vi "main.vi"() -> ()   [LabVIEW 2014]
uses:
  <vilib>/Instr/_visa.llb/VISA Configure Serial Port (Instr).vi
  <instrlib>/Keithley 24XX/Public/Data/Read (Single Point).vi
  <instrlib>/Keithley 24XX/Keithley 24XX.lvlib
panel:
  in  "Start Button":bool
  in  "Operation Mode":bool
  out "Humidity":sgl
  out "Humidity Data":string
  in  "Humidity Data":path=path "C:/Users/Administrator/Documents/humidity_sensing_setup/data/dumb/data_dumb_2.txt"
  out "Humidity Data Graph":sgl(graph)=5460.51
  out "Resistance Data":string
  in  "Resistance Data":path=path "C:/Users/Administrator/Documents/humidity_sensing_setup/data/dumb/data_dumb_1.txt"
  out "Current Data":string
  in  "Current Data":path=path "C:/Users/Administrator/Documents/humidity_sensing_setup/data/dumb/data_dumb.txt"
  in  "Sampling rate (ms/pt)":i32=1000
  in  "Stop Voltage/Current":dbl=1.0
  in  "Start Voltage/Current":dbl=1.0
  in  "current multiplier":dbl=1000000.0
  in  "stop button":bool
  out "Current Data Graph":sgl(graph)=0.0001831192
  out "Resistance Data Graph":sgl(graph)=5460.51
  in  "loop num":dbl=10000000000.0
  in  "Step":dbl
  in  "Source Mode  (0: Voltage)":u16(ring) items=["Voltage", "Current"]
  in  "Compliance  Level (0.1)":dbl=1.0
  in  "Enable Resistance Auto Range (T:Enable)":bool
  in  "Enable Current Auto Range (T:Enable)":bool=TRUE
  in  "Enable Voltage Auto Range (T:Enable)":bool
  in  "Resistance Manual Range (1.0)":dbl=1.0
  in  "Current Manual Range (1.0)":dbl=1.0
  in  "Voltage Manual Range (1.0)":dbl=1.0
  out "Resistance":sgl
  out "Current":sgl
  out "Voltage":sgl
  in  "Serial Configuration":T1={"Baud Rate"=9600, "Parity"=0, "Data Bits"=8, "Stop Bits"=10, "Flow Control"=0} {"Flow Control" items=["None", "XON/XOFF", "RTS/CTS", "XON/XOFF & RTS/CTS", "DTR/DSR", "XON/XOFF & DTR/DSR"]; "Stop Bits" items=["1.0"=10, "1.5"=15, "2.0"=20]; "Data Bits" items=["7"=7, "8"=8]; "Parity" items=["None", "Odd", "Even", "Mark", "Space"]; "Baud Rate" items=["300"=300, "600"=600, "1200"=1200, "2400"=2400, "4800"=4800, "9600"=9600, "19200"=19200]}
  in  "Keithley VISA resource name":refnum<visa-resource-name>="GPIB9::24::INSTR"
  out "Arduino Status":bool
  out "error out":errorcluster
  in  "error in":errorcluster
  in  "instr name":string="Arduino"
  in  "write":bool
  in  "buffer size":u32=256
  in  "timeout (ms)":u32=10000
  in  "flow control":u16
  in  "stop bits":u16=10
  in  "parity":u16(ring) items=["None", "Odd", "Even", "Mark", "Space"]
  in  "data bits":u16=8 min=5 max=8 step=1
  in  "baud rate":u32=9600
  in  "write string":string
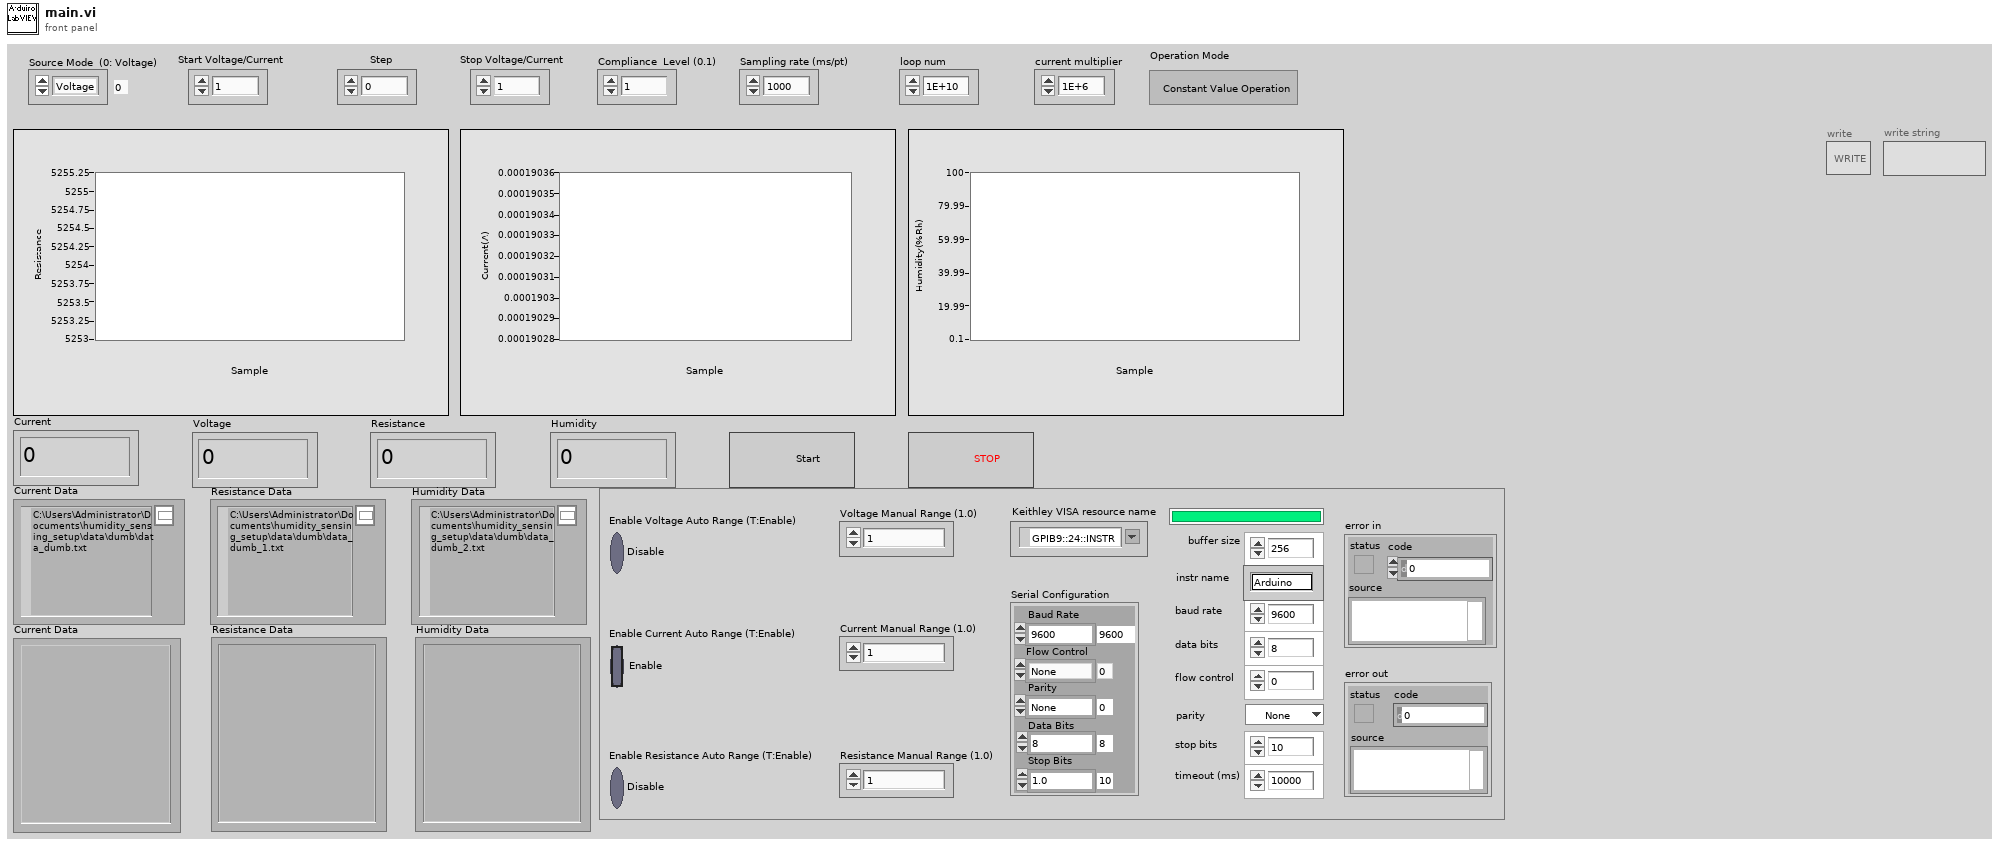
[diagram p1: front panel]
types:
  T1 = cluster{"Baud Rate":u32, "Parity":u16, "Data Bits":u16, "Stop Bits":u16, "Flow Control":u16}
  T2 = enum16{"open", "replace", "create", "open or create", "replace or create", "replace or create with confirmation"}
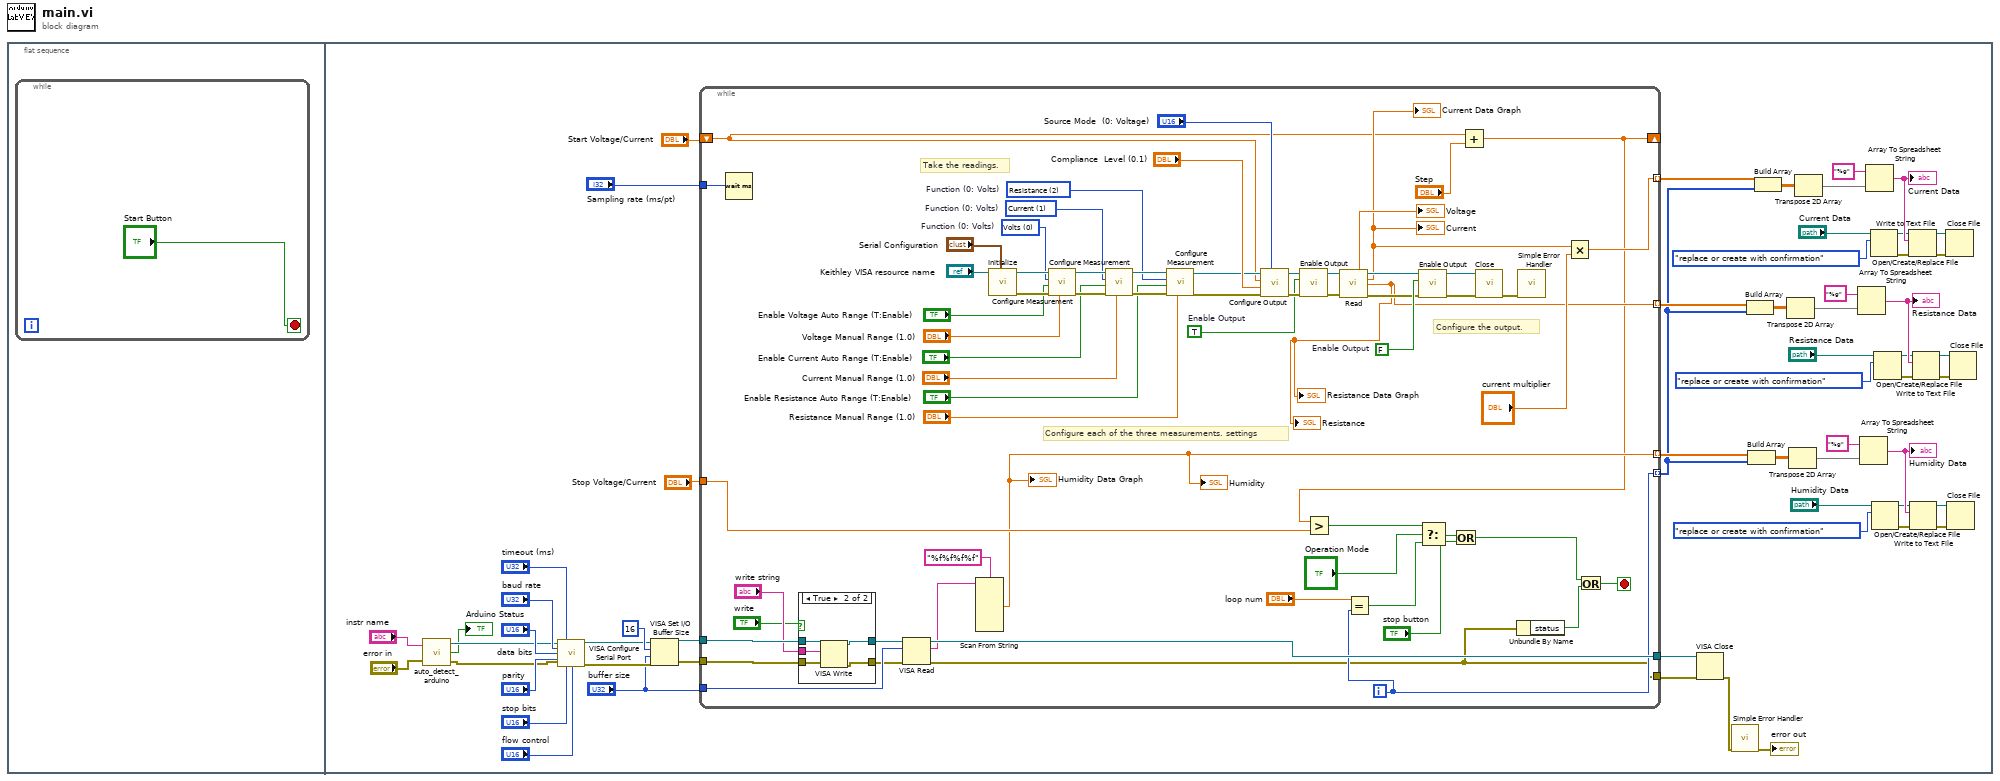
[diagram p0: block diagram]
diagram:
  n1 = flat-sequence {
    frame #0 {
      n2 = while {
        stop <- "Start Button" stop-if-true
      }
    }
    frame #1 {
      n3 = call "auto_detect_arduino.vi"("instr name"="instr name", "error in"="error in") -> ("VISA resource name"=w51:refnum<visa-resource-name>, "status"=→"Arduino Status":bool, "error out"=w50:errorcluster)
      n4 = call-poly "VISA Configure Serial Port"("VISA resource name"=w51, "timeout (10sec)"="timeout (ms)", "baud rate (9600)"="baud rate", "data bits (8)"="data bits", "parity (0:none)"="parity", "error in (no error)"=w50, "stop bits (10: 1 bit)"="stop bits", "flow control (0:none)"="flow control") -> ("VISA resource name out"=w47:refnum<visa-resource-name>, "error out"=w46:errorcluster)  [unwired: 6 in]
      n5 = VISA Set I/O Buffer Size(VISA resource name=w47, mask (16)=u16 16 ("I/O Receive\nBuffer mask"), size (4096)="buffer size", error in (no error)=w46) -> (VISA resource name out=w45:refnum<visa-resource-name>, error out=w44:errorcluster)
      n6 = while {
        tunnel: w45 -> [w120]
        tunnel: w44 -> [w119]
        tunnel: [w121] -> w59
        tunnel: [w63] -> w58
        tunnel: "buffer size" -> [w122]
        tunnel: [w65] -> w3 mode=indexing
        tunnel: "Sampling rate (ms/pt)" -> [w76]
        tunnel: "Stop Voltage/Current" -> [w75]
        tunnel: [w74] -> w16 mode=indexing
        tunnel: [w73] -> w2 mode=indexing
        tunnel: [w72] -> w15 mode=indexing
        shift-right: [w64] -> _
        shift-left: "Start Voltage/Current" -> [w71]
        i -> [w73]
        stop <- w123 stop-if-true
        w85 = TRUE  # Enable Output
        w95 = FALSE  # Enable Output
        w102 = u16 2 items=["Volts", "Current", "Resistance"]  # Function (0: Volts)
        w103 = u16 1 items=["Volts", "Current", "Resistance"]  # Function (0: Volts)
        w104 = u16 0 items=["Volts", "Current", "Resistance"]  # Function (0: Volts)
        # "Take the readings."
        # "Configure the output."
        # "Configure each of the three measurements. settings"
        n7 = Wait (ms)(milliseconds to wait=w76) -> ()  [unwired: 1 out]
        n8 = case shown="True" "write" {
          tunnel: w120 -> [w125 w130]
          tunnel: w119 -> [w124 w129]
          tunnel: [w125 w128] -> w118
          tunnel: [w124 w127] -> w117
          tunnel: "write string" -> [_ w126]
          frame False {
          }
          frame True {
            n9 = VISA Write(VISA resource name=w130, write buffer=w126, error in (no error)=w129) -> (VISA resource name out=w128:refnum<visa-resource-name>, error out=w127:errorcluster)  [unwired: 1 out]
          }
        }
        n10 = VISA Read(VISA resource name=w118, byte count=w122, error in (no error)=w117) -> (VISA resource name out=w121:refnum<visa-resource-name>, read buffer=w60:string, error out=w63:errorcluster)  [unwired: 1 out]
        n11 = Scan From String(format string="%f%f%f%f", input string=w60) -> (output 1=w65:sgl)  [unwired: 9 in, 3 out]
        "Humidity Data Graph" <- w65
        "Humidity" <- w65
        n12 = call <instrlib>:"Initialize.vi"("Serial Configuration"="Serial Configuration", "VISA resource name"="Keithley VISA resource name") -> ("error out"=w109:errorcluster, "VISA resource name out"=w110:refnum<visa-resource-name>)  [unwired: 8 in]
        n13 = call <instrlib>:"Configure Measurement.vi"("Manual Range (1.0)"="Voltage Manual Range (1.0)", "error in (no error)"=w109, "Enable Auto Range (T:Enable)"="Enable Voltage Auto Range (T:Enable)", "Function (0: Volts)"=w104, "VISA resource name"=w110) -> ("error out"=w107:errorcluster, "VISA resource name out"=w108:refnum<visa-resource-name>)  [unwired: 5 in]
        n14 = call <instrlib>:"Configure Measurement.vi"("Manual Range (1.0)"="Current Manual Range (1.0)", "error in (no error)"=w107, "Enable Auto Range (T:Enable)"="Enable Current Auto Range (T:Enable)", "Function (0: Volts)"=w103, "VISA resource name"=w108) -> ("error out"=w106:errorcluster, "VISA resource name out"=w105:refnum<visa-resource-name>)  [unwired: 5 in]
        n15 = call <instrlib>:"Configure Measurement.vi"("Manual Range (1.0)"="Resistance Manual Range (1.0)", "error in (no error)"=w106, "Enable Auto Range (T:Enable)"="Enable Resistance Auto Range (T:Enable)", "Function (0: Volts)"=w102, "VISA resource name"=w105) -> ("error out"=w84:errorcluster, "VISA resource name out"=w83:refnum<visa-resource-name>)  [unwired: 5 in]
        n16 = call <instrlib>:"Configure Output.vi"("Source Mode  (0: Voltage)"="Source Mode  (0: Voltage)", "error in (no error)"=w84, "Compliance  Level (0.1)"="Compliance  Level (0.1)", "Output Level (0)"=w71, "VISA resource name"=w83) -> ("error out"=w86:errorcluster, "VISA resource name out"=w87:refnum<visa-resource-name>)  [unwired: 5 in]
        n17 = call <instrlib>:"Enable Output.vi"("error in (no error)"=w86, "Enable Output (T: Enable)"=w85, "VISA resource name"=w87) -> ("error out"=w89:errorcluster, "VISA resource name out"=w88:refnum<visa-resource-name>)  [unwired: 7 in]
        n18 = call-poly <instrlib>:"Read.vi"("VISA resource name"=w88, "error in (no error)"=w89) -> ("Voltage"=→"Voltage":sgl, "VISA resource name out"=w90:refnum<visa-resource-name>, "Current"=w78:sgl, "Resistance"=w72:sgl, "error out"=w91:errorcluster)  [unwired: 7 in, 2 out]
        "Current" <- w78
        "Resistance" <- w72
        "Resistance Data Graph" <- w72
        "Current Data Graph" <- w78
        n19 = Equal?(x="loop num", y=w73) -> (x = y?=w66:bool)
        n20 = call <instrlib>:"Enable Output.vi"("error in (no error)"=w91, "Enable Output (T: Enable)"=w95, "VISA resource name"=w90) -> ("error out"=w92:errorcluster, "VISA resource name out"=w93:refnum<visa-resource-name>)  [unwired: 7 in]
        n21 = Add(x=w71, y="Step") -> (x+y=w64:dbl)
        n22 = Greater?(x=w64, y=w75) -> (0:w69:bool)
        n23 = Select(t=w69, s="Operation Mode", f=w66) -> (s? t:f=w68:bool)
        n24 = Or(x=w68, y="stop button") -> (x .or. y?=w61:bool)
        n25 = call <instrlib>:"Close.vi"("error in (no error)"=w92, "VISA resource name"=w93) -> ("error out"=w113:errorcluster)  [unwired: 9 in]
        n26 = Unbundle By Name(w63) -> ("status"=w62:bool)
        n27 = call <vilib>:"Simple Error Handler.vi"("error in (no error)"=w113) -> ()  [unwired: 4 in, 5 out]
        n28 = Multiply(x=w78, y="current multiplier") -> (x*y=w74:dbl)
        n29 = Or(x=w61, y=w62) -> (x .or. y?=w123:bool)
      }
      n30 = VISA Close(VISA resource name=w59, error in (no error)=w58) -> (error out=w41:errorcluster)
      n31 = call <vilib>:"Simple Error Handler.vi"("error in (no error)"=w41) -> ("error out"=→"error out":errorcluster)  [unwired: 4 in, 4 out]
      n32 = Build Array(w15, w2) -> (w17:sgl[][])
      n33 = Build Array(w3, w2) -> (w4:sgl[][])
      n34 = Build Array(w16, w2) -> (w33:dbl[][])
      n35 = Transpose 2D Array(2D array=w17) -> (transposed array=w25:sgl[][])
      n36 = Transpose 2D Array(2D array=w4) -> (transposed array=w12:sgl[][])
      n37 = Transpose 2D Array(2D array=w33) -> (transposed array=w35:dbl[][])
      n38 = Array To Spreadsheet String(array=w25, 3:"%g" ("format string")) -> (spreadsheet string=w26:string)  [unwired: 1 in]
      "Resistance Data" <- w26
      n39 = Array To Spreadsheet String(array=w12, 3:"%g" ("format string")) -> (spreadsheet string=w13:string)  [unwired: 1 in]
      "Humidity Data" <- w13
      n40 = Array To Spreadsheet String(array=w35, 3:"%g" ("format string")) -> (spreadsheet string=w36:string)  [unwired: 1 in]
      "Current Data" <- w36
      n41 = Open/Create/Replace File(file path (use dialog)="Current Data", operation (0:open)=T2."replace or create with confirmation") -> (refnum out=w32:refnum<file>, error out=w27:errorcluster)  [unwired: 4 in, 1 out]
      n42 = Open/Create/Replace File(file path (use dialog)="Humidity Data", operation (0:open)=T2."replace or create with confirmation") -> (refnum out=w10:refnum<file>, error out=w5:errorcluster)  [unwired: 4 in, 1 out]
      n43 = Open/Create/Replace File(file path (use dialog)="Resistance Data", operation (0:open)=T2."replace or create with confirmation") -> (refnum out=w23:refnum<file>, error out=w18:errorcluster)  [unwired: 4 in, 1 out]
      n44 = Write to Text File(file (use dialog)=w32, text=w36, error in=w27) -> (refnum out=w29:refnum<file>, error out=w28:errorcluster)  [unwired: 2 out]
      n45 = Write to Text File(file (use dialog)=w10, text=w13, error in=w5) -> (refnum out=w7:refnum<file>, error out=w6:errorcluster)  [unwired: 2 out]
      n46 = Write to Text File(file (use dialog)=w23, text=w26, error in=w18) -> (refnum out=w20:refnum<file>, error out=w19:errorcluster)  [unwired: 2 out]
      n47 = Close File(refnum=w29, error in=w28) -> ()  [unwired: 2 out]
      n48 = Close File(refnum=w7, error in=w6) -> ()  [unwired: 2 out]
      n49 = Close File(refnum=w20, error in=w19) -> ()  [unwired: 2 out]
    }
  }
